vi "PoseAndTargeting.vi"() -> ()   [LabVIEW 2020]
doc: "Manages the robot's pose (position, heading, and velocity) and targeting information. Data from the IMU, swerve drive encoders, swerve azimuth encoders, turret enoder, and LimeLight are fused together to estimate these values. Supports pose resets on boot, from the Autonomous Sequencer, and on command from the FRC 4265 Dashboard."
uses:
  GlobalDrivebase.vi
panel:
  in  "Max Vision X (in)":dbl=100.0
  in  "Min Timed Aligned (ms)":u32=200
  in  "Acceptable Heading Error (deg)":dbl=5.0
  in  "Vision Trust Threshold (in)":dbl=10.0
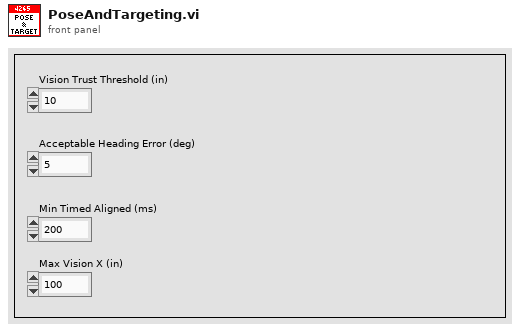
[diagram p1: front panel]
types:
  T1 = cluster{"Transitioning":bool, "Position (in)":dbl, "Velocity (ft/s)":dbl, "Azimuth Position (deg) [-180,+180]":dbl}
  T2 = enum16{"Normal", "Auto Set", "Reset IMU", "Manual Push", "Init"}
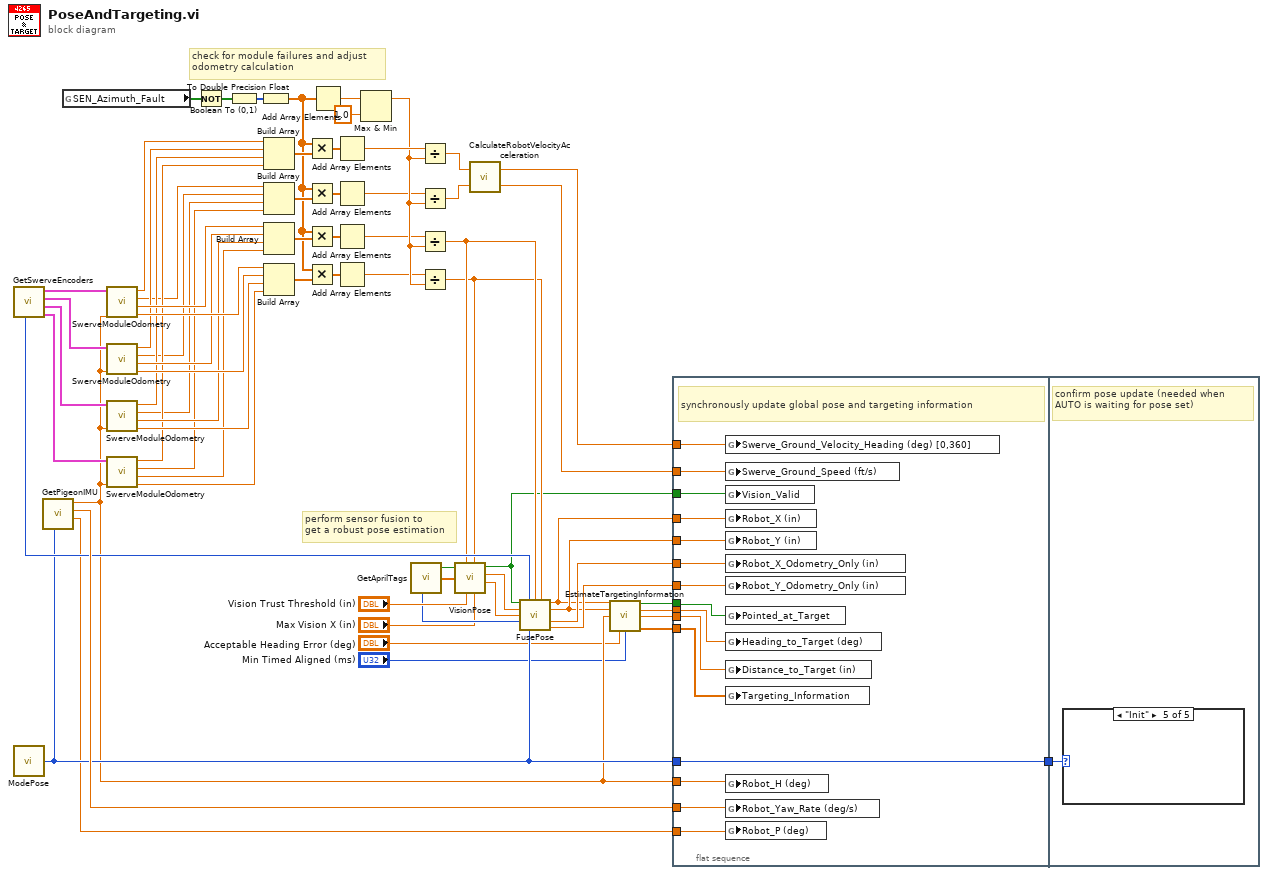
[diagram p0: block diagram]
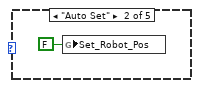
[diagram p3: hidden frame]
diagram:
  # "perform sensor fusion to\nget a robust pose estimation"
  # "check for module failures and adjust\nodometry calculation"
  n1 = call "GetSwerveEncoders.vi"() -> ("Swerve 3 Encoder Data"=w24:T1, "Swerve 2 Encoder Data"=w25:T1, "Swerve 1 Encoder Data"=w26:T1, "Swerve 0 Encoder Data"=w27:T1, "Odometry Timestamp (ms)"=w22:u32)  [unwired: 5 in]
  n2 = call "ModePose.vi"() -> ("Pose Mode"=w12:T2)  [unwired: 1 in]
  n3 = call "GetPigeonIMU.vi"("Pose Mode"=w12) -> ("Yaw (deg)"=w11:dbl, "Yaw Rate (deg/s)"=w49:dbl, "Pitch (deg)"=w6:dbl)  [unwired: 5 in]
  n4 = global read "GlobalDrivebase.vi" "SEN_Azimuth_Fault"() -> (w38:bool[])
  n5 = call "SwerveModuleOdometry.vi"("Robot Heading(deg)"=w11, "Swerve Encoder Data"=w27) -> ("Delta Y (in)"=w66:dbl, "Delta X (in)"=w65:dbl, "Velocity Y (ft/s)"=w58:dbl, "Velocity X (ft/s)"=w45:dbl)  [unwired: 4 in]
  n6 = call "SwerveModuleOdometry.vi"("Robot Heading(deg)"=w11, "Swerve Encoder Data"=w26) -> ("Delta Y (in)"=w67:dbl, "Delta X (in)"=w64:dbl, "Velocity Y (ft/s)"=w57:dbl, "Velocity X (ft/s)"=w61:dbl)  [unwired: 4 in]
  n7 = call "SwerveModuleOdometry.vi"("Robot Heading(deg)"=w11, "Swerve Encoder Data"=w25) -> ("Delta Y (in)"=w68:dbl, "Delta X (in)"=w63:dbl, "Velocity Y (ft/s)"=w56:dbl, "Velocity X (ft/s)"=w60:dbl)  [unwired: 4 in]
  n8 = call "SwerveModuleOdometry.vi"("Robot Heading(deg)"=w11, "Swerve Encoder Data"=w24) -> ("Delta Y (in)"=w69:dbl, "Delta X (in)"=w62:dbl, "Velocity Y (ft/s)"=w55:dbl, "Velocity X (ft/s)"=w59:dbl)  [unwired: 4 in]
  n9 = Not(x=w38) -> (.not. x?=w47:bool[])
  n10 = Boolean To (0,1)(Boolean=w47) -> (0, 1=w46:i16[])
  n11 = To Double Precision Float(number=w46) -> (double precision float=w29:dbl[])
  n12 = Build Array(w45, w61, w60, w59) -> (w39:dbl[])
  n13 = Build Array(w58, w57, w56, w55) -> (w36:dbl[])
  n14 = Build Array(w65, w64, w63, w62) -> (w33:dbl[])
  n15 = Build Array(w66, w67, w68, w69) -> (w30:dbl[])
  n16 = Multiply(x=w29, y=w39) -> (x*y=w44:dbl[])
  n17 = Multiply(x=w29, y=w36) -> (x*y=w37:dbl[])
  n18 = Multiply(x=w29, y=w33) -> (x*y=w34:dbl[])
  n19 = Multiply(x=w29, y=w30) -> (x*y=w31:dbl[])
  n20 = Add Array Elements(numeric array=w29) -> (sum=w42:dbl)
  n21 = Add Array Elements(numeric array=w44) -> (sum=w43:dbl)
  n22 = Add Array Elements(numeric array=w37) -> (sum=w35:dbl)
  n23 = Add Array Elements(numeric array=w34) -> (sum=w32:dbl)
  n24 = Add Array Elements(numeric array=w31) -> (sum=w28:dbl)
  n25 = Max & Min(x=w42, y=1.0) -> (max(x,y)=w40:dbl)  [unwired: 1 out]
  n26 = call "GetAprilTags.vi"() -> ("Vision Timestamp (ms)"=w16:u32, "Vision Target Valid [t-?]"=w54:bool, "AprilTag Data [t-?]"=w23:dbl[])  [unwired: 6 in]
  n27 = Divide(x=w43, y=w40) -> (x/y=w52:dbl)
  n28 = Divide(x=w35, y=w40) -> (x/y=w53:dbl)
  n29 = Divide(x=w32, y=w40) -> (x/y=w21:dbl)
  n30 = Divide(x=w28, y=w40) -> (x/y=w20:dbl)
  n31 = call "VisionPose.vi"("Max Vision X (in)"="Max Vision X (in)", "Odometry Delta Y (in) [t0]"=w20, "Vision Trust Threshold (in)"="Vision Trust Threshold (in)", "Odometry Delta X (in) [t0]"=w21, "AprilTag Data [t-?]"=w23, "Vision Target Valid [t-?]"=w54) -> ("Vision Y (in) [t-?]"=w17:dbl, "Vision X (in) [t-?]"=w18:dbl, "Vision Valid [t-?]"=w19:bool)  [unwired: 3 in]
  n32 = call "CalculateRobotVelocityAcceleration.vi"("Velocity Y (ft/s)"=w53, "Velocity X (ft/s)"=w52) -> ("Velocity Magnitude (ft/s)"=w51:dbl, "Velocity Heading (deg)"=w50:dbl)
  n33 = call "FusePose.vi"("Vision Valid [t-?]"=w19, "Odometry Timestamp (ms)"=w22, "Odometry Delta X (in) [t0]"=w21, "Odometry Delta Y (in) [t0]"=w20, "Vision X (in) [t-?]"=w18, "Vision Y (in) [t-?]"=w17, "Vision Timestamp (ms)"=w16, "Pose Mode"=w12) -> ("X (in) [t0]"=w1:dbl, "Y (in) [t0]"=w2:dbl, "X Odometry Only (in) [t0]"=w15:dbl, "Y Odometry Only (in) [t0]"=w14:dbl)  [unwired: 4 in]
  n34 = call "EstimateTargetingInformation.vi"("X (in) [t0]"=w1, "Y (in) [t0]"=w2, "Robot Heading (deg)"=w11, "Acceptable Heading Error (deg)"="Acceptable Heading Error (deg)", "Min Timed Aligned (ms)"="Min Timed Aligned (ms)") -> ("Pointed At Target"=w10:bool, "Heading to Target (deg)"=w9:dbl, "Distance to Target (in)"=w8:dbl, "Targeting Information"=w7:dbl[])  [unwired: 7 in]
  n35 = flat-sequence {
    tunnel: w11 -> [w84]
    tunnel: w19 -> [w83]
    tunnel: w51 -> [w82]
    tunnel: w50 -> [w81]
    tunnel: w49 -> [w80]
    tunnel: w1 -> [w79]
    tunnel: w2 -> [w78]
    tunnel: w15 -> [w77]
    tunnel: w14 -> [w76]
    tunnel: w12 -> [w75]
    tunnel: [w75] -> w13
    tunnel: w10 -> [w72]
    tunnel: w9 -> [w71]
    tunnel: w8 -> [w70]
    tunnel: w7 -> [w74]
    tunnel: w6 -> [w73]
    tunnel: w13 -> [w85]
    frame #0 {
      # "synchronously update global pose and targeting information"
      n36 = global write "GlobalPoseAndTargeting.vi" "Swerve_Ground_Velocity_Heading (deg) [0,360]"(w81) -> ()
      n37 = global write "GlobalPoseAndTargeting.vi" "Swerve_Ground_Speed (ft/s)"(w82) -> ()
      n38 = global write "GlobalPoseAndTargeting.vi" "Vision_Valid"(w83) -> ()
      n39 = global write "GlobalPoseAndTargeting.vi" "Robot_X (in)"(w79) -> ()
      n40 = global write "GlobalPoseAndTargeting.vi" "Robot_Y (in)"(w78) -> ()
      n41 = global write "GlobalPoseAndTargeting.vi" "Robot_X_Odometry_Only (in)"(w77) -> ()
      n42 = global write "GlobalPoseAndTargeting.vi" "Robot_Y_Odometry_Only (in)"(w76) -> ()
      n43 = global write "GlobalPoseAndTargeting.vi" "Pointed_at_Target"(w72) -> ()
      n44 = global write "GlobalPoseAndTargeting.vi" "Heading_to_Target (deg)"(w71) -> ()
      n45 = global write "GlobalPoseAndTargeting.vi" "Distance_to_Target (in)"(w70) -> ()
      n46 = global write "GlobalPoseAndTargeting.vi" "Targeting_Information"(w74) -> ()
      n47 = global write "GlobalPoseAndTargeting.vi" "Robot_H (deg)"(w84) -> ()
      n48 = global write "GlobalPoseAndTargeting.vi" "Robot_Yaw_Rate (deg/s)"(w80) -> ()
      n49 = global write "GlobalPoseAndTargeting.vi" "Robot_P (deg)"(w73) -> ()
    }
    frame #1 {
      # "confirm pose update (needed when AUTO is waiting for pose set)"
      n50 = case shown="\"Init\"" w85 {
        frame "Normal", Default {
        }
        frame "Auto Set" {
          n51 = global write "GlobalPoseAndTargeting.vi" "Set_Robot_Pos"(FALSE ("Set_Robot_Pos")) -> ()
        }
        frame "Reset IMU" {
        }
        frame "Manual Push" {
        }
        frame "Init" {
        }
      }
    }
  }
